vi "Read Input queue.vi"(8 "error in (no error)":errorcluster, 11 "BaseDriver in":refnum<class "BaseDriver.lvclass">) -> (0 "error out":errorcluster, 2 "Message queue":T1, 3 "BaseDriver out":refnum<class "BaseDriver.lvclass">)   [LabVIEW 2013, in "BaseDriver.lvclass"]
doc: "Use the input queue to send messages to the driver. It will interprete the messages and if transmit them to the remote destination"
uses:
  BaseDriver.lvclass
  message_queue.ctl
  Message/BaseMessage/BaseMessage.lvclass
  BaseDriver.lvclass/BaseDriver.ctl
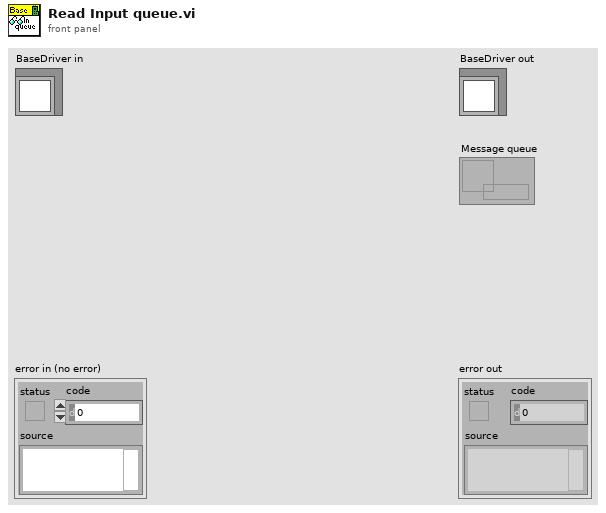
[diagram p1: front panel]
types:
  T1 = typedef "message_queue.ctl" = refnum<queue>
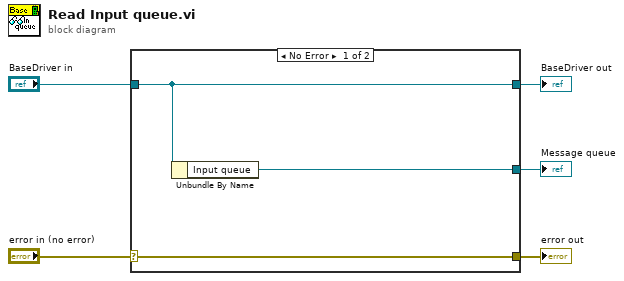
[diagram p0: block diagram]
diagram:
  n1 = case shown="No Error" "error in (no error)" {
    selector: "error in (no error)" -> [w8 w9]
    tunnel: [w8 w9] -> w4
    tunnel: [w7 w10] -> w2
    tunnel: "BaseDriver in" -> [w7 w10]
    tunnel: [w6 _] -> w1
    frame No Error {
      n2 = Unbundle By Name(w7) -> ("Input queue"=w6:T1)
    }
    frame Error {
    }
  }
  "error out" <- w4
  "BaseDriver out" <- w2
  "Message queue" <- w1
